vi "preprocessing.vi"(7 "WaveformGraph in":refnum<vi>, 9 "Input Speech":waveform(dbl)[](graph)) -> (1 "Start index":dbl, 2 "Frames":dbl[][](array[numeric]), 3 "Signal energy":dbl, 4 "Boolean":bool)   [LabVIEW 2013]
uses:
  <vilib>/Analysis/3filter.llb/FIR Filter (DBL).vi
  <vilib>/Analysis/NI_AALBase.lvlib
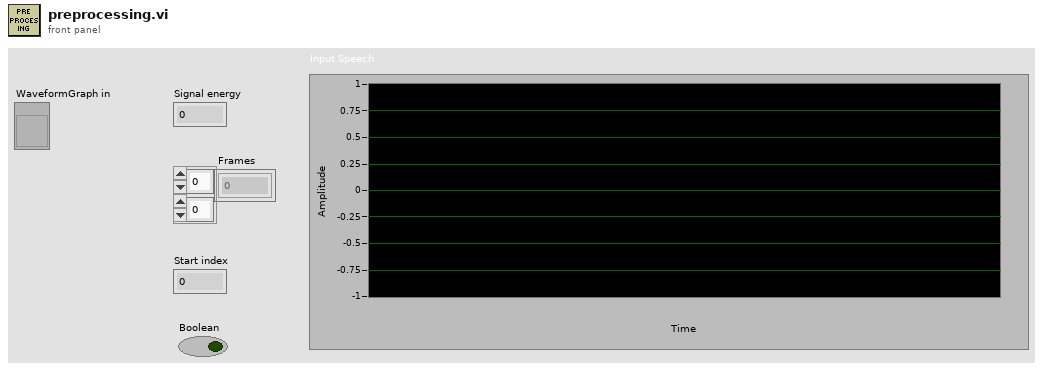
[diagram p1: front panel]
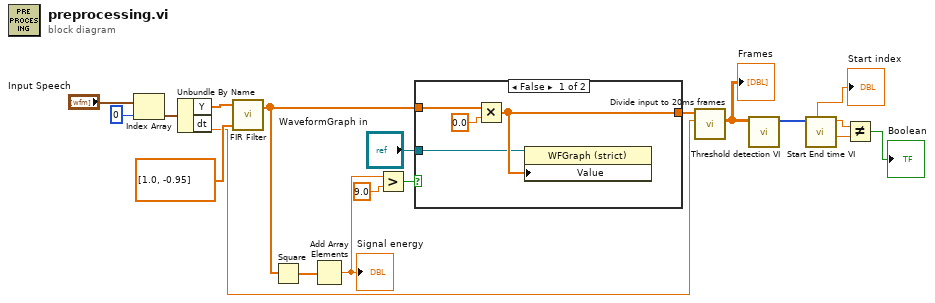
[diagram p0: block diagram]
diagram:
  n1 = Index Array(array="Input Speech", index=0) -> (element=w4:waveform(dbl))
  n2 = Unbundle By Name(w4) -> ("Y"=w2:dbl[], "dt"=w1:dbl)
  n3 = call-poly <vilib>:"FIR Filter.vi"("FIR Coefficients"=dbl[] [1.0, -0.95], "X"=w2) -> ("Filtered X"=w18:dbl[])  [unwired: 2 in, 1 out]
  n4 = Square(x=w18) -> (x^2=w14:dbl[])
  n5 = Add Array Elements(numeric array=w14) -> (sum=w16:dbl)
  "Signal energy" <- w16
  n6 = Greater?(x=w16, y=9.0) -> (0:w17:bool)
  n7 = case shown="False" w17 {
    tunnel: w18 -> [w22 w24]
    tunnel: [w21 w24] -> w19
    tunnel: "WaveformGraph in" -> [w20 _]
    frame False {
      n8 = Multiply(x=w22, y=0.0) -> (x*y=w21:dbl[])
      n9 = property class="WFGraph (strict)"(reference=w20, "Value"=w21) -> ()  [unwired: 1 in, 2 out]
    }
    frame True {
    }
  }
  n10 = call "Divide input to 20ms frames.vi"("dt"=w1, "Y"=w19) -> ("Frames Matrix"=w12:dbl[][])  [unwired: 6 in, 3 out]
  "Frames" <- w12
  n11 = call "Threshold detection VI.vi"("Windowed Frames"=w12) -> ("Boolean frame energy"=w7:i16[])  [unwired: 8 in, 2 out]
  n12 = call "Start End time VI.vi"("Boolean frame energy"=w7) -> ("End Time"=w8:dbl, "Start Time"=w9:dbl, "min index"=→"Start index":dbl)  [unwired: 5 in, 3 out]
  n13 = Not Equal?(x=w9, y=w8) -> (x != y?=→"Boolean":bool)
